vi "MoveNode.vi"(8 "error in":errorcluster, 10 "new parent":T1, 11 "node":T1) -> (0 "error out":errorcluster)   [LabVIEW 2013, in "NISE_CEF_TreeControl.lvlib"]
doc: "Moves a node to a new parretn updating the reference in the 3 nodes (child, old parent and new parent)."
uses:
  NISE_CEF_TreeControl.lvlib
  Node/NodeRef.ctl
  Node/NISE_CEF_Node.lvclass
  Node/NISE_CEF_Node.lvclass/NISE_CEF_Node.ctl
  Node/ReadParent.vi
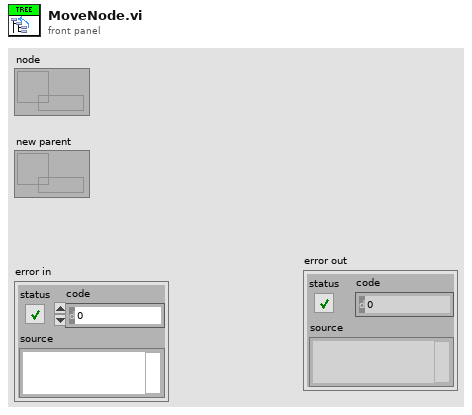
[diagram p1: front panel]
types:
  T1 = typedef "NISE_CEF_Node.lvclass/NodeRef.ctl" = refnum<data-value>
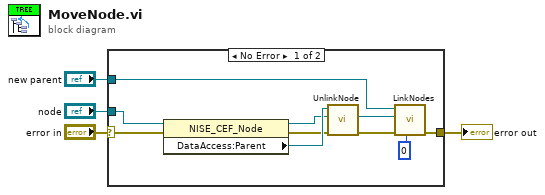
[diagram p0: block diagram]
diagram:
  n1 = case shown="No Error" "error in" {
    selector: "error in" -> [w6 w15]
    tunnel: [w8 w15] -> w3
    tunnel: "node" -> [w13 _]
    tunnel: "new parent" -> [w9 _]
    frame No Error {
      n2 = property class="NISE_CEF_Node"(reference=w13, error in=w6) -> (reference out=w10:T1, error out=w7:errorcluster, "DataAccess:Parent"=w14:T1)
      n3 = call "UnlinkNode.vi"("error in"=w7, "child in"=w10, "parent in"=w14) -> ("error out"=w12:errorcluster, "child out"=w11:T1)  [unwired: 6 in, 1 out]
      n4 = call "LinkNodes.vi"("index"=0, "error in"=w12, "child in"=w11, "parent in"=w9) -> ("error out"=w8:errorcluster)  [unwired: 5 in, 2 out]
    }
    frame Error {
    }
  }
  "error out" <- w3
